vi "MGCC_StaEst_load_complex.vi"(1 "file path (dialog if empty)":path) -> (0 "Array 13":cdb[][](array[numeric]))   [LabVIEW 2016]
uses:
  <vilib>/Utility/file.llb/Read Delimited Spreadsheet (string).vi
panel:
  out "error out":errorcluster
  in  "Array 12":cdb[][](array[numeric])
  out "all rows":string[][](array[string])
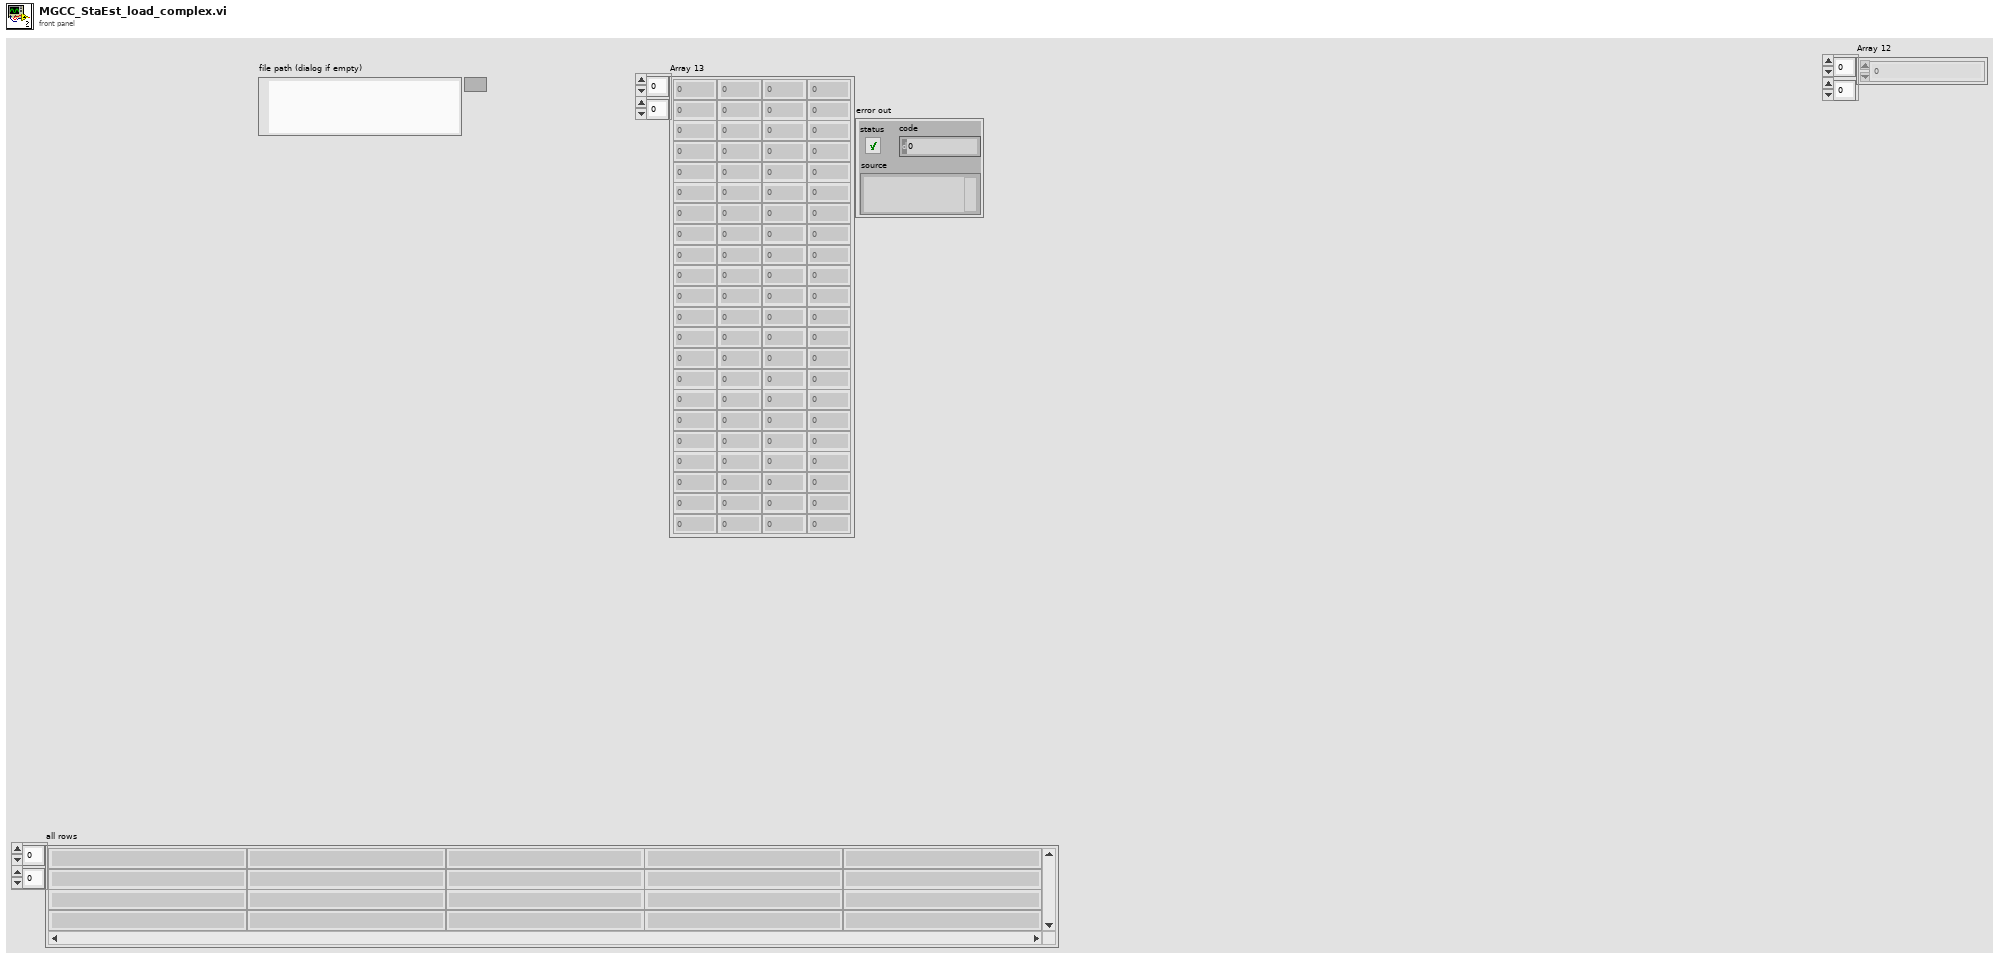
[diagram p1: front panel]
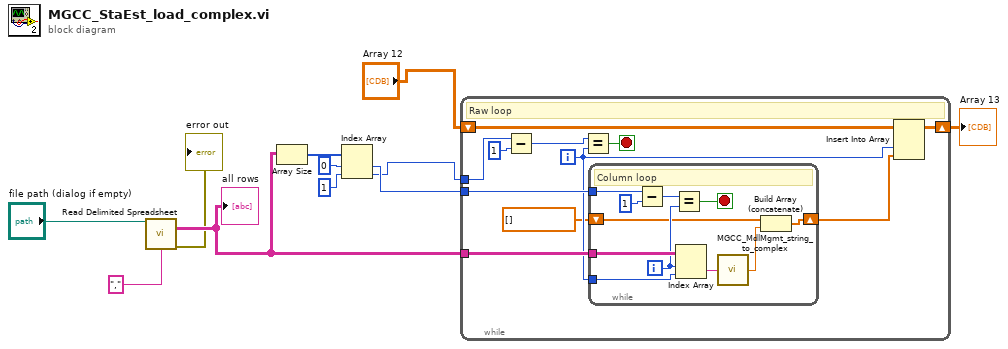
[diagram p0: block diagram]
diagram:
  n1 = call-poly <vilib>:"Read Delimited Spreadsheet.vi"("file path (dialog if empty)"="file path (dialog if empty)", "delimiter (\\t)"="," ("delimiter (\\t)")) -> ("all rows"=w7:string[][], "error out"=→"error out":errorcluster)  [unwired: 8 in, 4 out]
  "all rows" <- w7
  n2 = Array Size(array=w7) -> (size(s)=w11:i32[])
  n3 = Index Array(array=w11, index #1=0 ("index"), index #2=1 ("index")) -> (element #1=w9:i32, element #2=w5:i32)
  n4 = while {
    tunnel: w7 -> [w22]
    tunnel: w9 -> [w21]
    tunnel: w5 -> [w19]
    shift-right: [w15] -> w3
    shift-left: "Array 12" -> [w16]
    i -> [w14]
    stop <- w17 stop-if-true
    # "Raw loop"
    n5 = Subtract(x=w19, y=1) -> (x-y=w18:i32)
    n6 = Equal?(x=w18, y=w14) -> (x = y?=w17:bool)
    n7 = while {
      tunnel: w22 -> [w31]
      tunnel: w21 -> [w28]
      shift-right: [w23] -> w13
      shift-left: cdb[] [] -> [w29]
      tunnel: w14 -> [w24]
      i -> [w30]
      stop <- w33 stop-if-true
      # "Column loop"
      n8 = Subtract(x=w28, y=1) -> (x-y=w26:i32)
      n9 = Equal?(x=w26, y=w30) -> (x = y?=w33:bool)
      n10 = Index Array(array=w31, index (row)=w30, index (col)=w24) -> (element=w25:string)
      n11 = call "MGCC_MdlMgmt_string_to_complex.vi"("String Input"=w25) -> ("Complex Number"=w32:cdb)
      n12 = Build Array (concatenate)(w29, w32) -> (w23:cdb[])
    }
    n13 = Insert Into Array(array=w16, index (col)=w14, new element=w13) -> (w15:cdb[][])  [unwired: 1 in]
  }
  "Array 13" <- w3
